vi "test1.vi"() -> ()   [LabVIEW 2020]
uses:
  Control 1.ctl
panel:
  in  "Stop":bool
  out "Message":string
  in  "Hello":bool
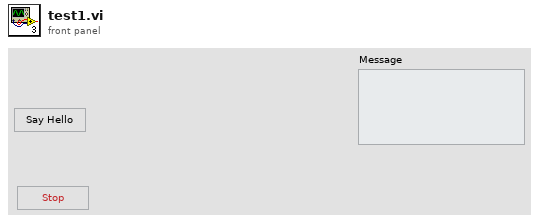
[diagram p1: front panel]
types:
  T1 = typedef "Control 1.ctl" = enum16{"Init", "Hello", "Stop"}
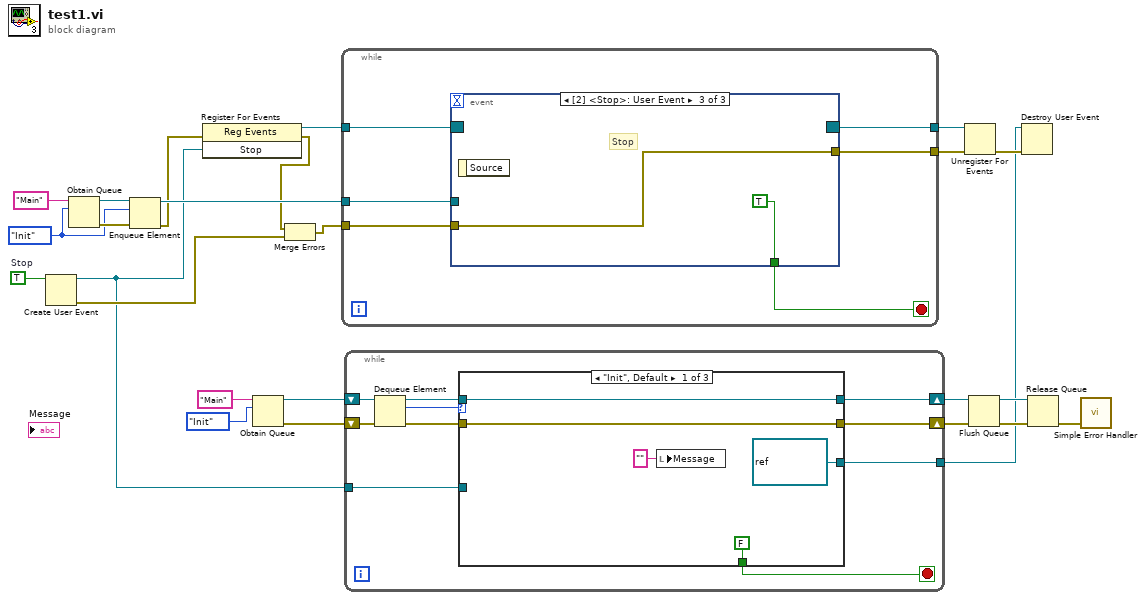
[diagram p0: block diagram]
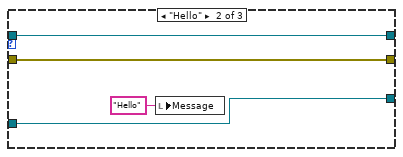
[diagram p2: hidden frame]
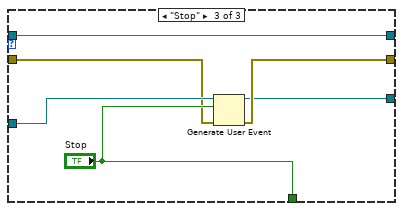
[diagram p3: hidden frame]
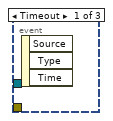
[diagram p4: hidden frame]
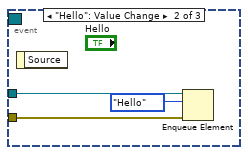
[diagram p5: hidden frame]
diagram:
  w6 = TRUE  # Stop
  w16 = Control_1."Init"
  n1 = Create User Event(user event datatype=w6) -> (user event=w2:refnum<user-event>, error out=w17:errorcluster)  [unwired: 1 in]
  n2 = Obtain Queue(name (unnamed)="Main", element data type=w16) -> (queue out=w22:refnum<queue>, error out=w24:errorcluster)  [unwired: 3 in, 1 out]
  n3 = Enqueue Element(queue=w22, element=w16, error in (no error)=w24) -> (queue out=w23:refnum<queue>, error out=w19:errorcluster)  [unwired: 1 in, 1 out]
  n4 = register-events(error in=w19, w2) -> (reference out=w21:refnum<event-registration>, error out=w18:errorcluster)  [unwired: 1 in]
  n5 = Obtain Queue(name (unnamed)="Main", element data type=Control_1."Init") -> (queue out=w13:refnum<queue>, error out=w12:errorcluster)  [unwired: 3 in, 1 out]
  n6 = Merge Errors(w18, w17) -> (w20:errorcluster)
  n7 = while {
    tunnel: w20 -> [w31]
    tunnel: w23 -> [w30]
    tunnel: w21 -> [w29]
    tunnel: [w27] -> w4
    tunnel: [w26] -> w5
    stop <- w28 stop-if-true
    n8 = event shown="[2] <Stop>: User Event" {
      selector: w29 -> [_ _ _]
      dyn-events: [_ _ _] -> w27
      timeout: _ -> [_ _ _]
      tunnel: w31 -> [_ w33 w35]
      tunnel: w30 -> [_ w34 _]
      tunnel: [_ _ TRUE] -> w28
      tunnel: [_ _ w35] -> w26
      event Timeout {
        n9 = event-data() -> ()  [unwired: 1 in, 3 out]
      }
      event "Hello": Value Change {
        n10 = event-data() -> ()  [unwired: 1 in, 1 out]
        n11 = Enqueue Element(queue=w34, element=Control_1."Hello", error in (no error)=w33) -> ()  [unwired: 1 in, 3 out]
      }
      event User Event {
        # "Stop"
        n12 = event-data() -> ()  [unwired: 1 in, 1 out]
      }
    }
  }
  n13 = while {
    tunnel: w2 -> [w38]
    shift-right: [w40] -> w11
    shift-left: w13 -> [w46]
    shift-right: [w39] -> w10
    shift-left: w12 -> [w45]
    tunnel: [w37] -> w1
    stop <- w41 stop-if-true
    n14 = Dequeue Element(queue=w46, error in (no error)=w45) -> (queue out=w44:refnum<queue>, element=w42:T1, error out=w43:errorcluster)  [unwired: 1 in, 1 out]
    n15 = case shown="\"Init\", Default" w42 {
      tunnel: w44 -> [w50 w54 w61]
      tunnel: w43 -> [w49 w53 w58]
      tunnel: [FALSE ("Stop") _ "Stop"] -> w41
      tunnel: [w50 w54 w61] -> w40
      tunnel: [w49 w53 w57] -> w39
      tunnel: w38 -> [_ w52 w60]
      tunnel: [refnum<user-event> refnum ("Stop") w52 w56] -> w37
      frame "Init", Default {
        n16 = local write "Message"("" ("Message")) -> ()
      }
      frame "Hello" {
        n17 = local write "Message"("Hello" ("Message")) -> ()
      }
      frame "Stop" {
        n18 = Generate User Event(user event=w60, event data cluster="Stop", error in=w58) -> (user event out=w56:refnum<user-event>, error out=w57:errorcluster)  [unwired: 1 in]
      }
    }
  }
  n19 = Unregister For Events(event registration refnum=w4, error in=w5) -> (error out=w3:errorcluster)
  n20 = Flush Queue(queue=w11, error in (no error)=w10) -> (queue out=w8:refnum<queue>, error out=w9:errorcluster)  [unwired: 1 out]
  n21 = Destroy User Event(user event=w1, error in=w3) -> ()  [unwired: 1 out]
  n22 = Release Queue(queue=w8, error in (no error)=w9) -> (error out=w7:errorcluster)  [unwired: 1 in, 2 out]
  n23 = call <vilib>:"Simple Error Handler.vi"("error in (no error)"=w7) -> ()  [unwired: 4 in, 5 out]
